vi "Test3.vi"() -> ()   [LabVIEW 2012]
uses:
  <vilib>/Rock Robotics/SystemInterfaces/DIO/FPGA_DIOChannel.ctl
  <vilib>/Rock Robotics/SystemInterfaces/DIO/FPGA_DIORelayChannel.ctl
  <vilib>/Rock Robotics/WPI/Solenoid/WPI_SolenoidChannel.ctl
  <vilib>/Rock Robotics/SystemInterfaces/Typedef/FPGA_TypedefSolenoidModule.ctl
  <vilib>/Rock Robotics/WPI/Solenoid/WPI_SolenoidValue.ctl
  <vilib>/Rock Robotics/WPI/Solenoid/WPI_SolenoidOpenDouble.vi
  <vilib>/Rock Robotics/WPI/Joystick/WPI_JoystickGetSetRefNum.vi
  <vilib>/Rock Robotics/WPI/Solenoid/WPI_SolenoidSetEnum.vi
panel:
  in  "TeleOp Elapsed Seconds":dbl
  in  "stop 2":bool
  in  "S On Time":dbl
  in  "S Off Time":dbl
  in  "stop":bool
  in  "Ready To Fire":bool
  out "Time Last Fired":dbl
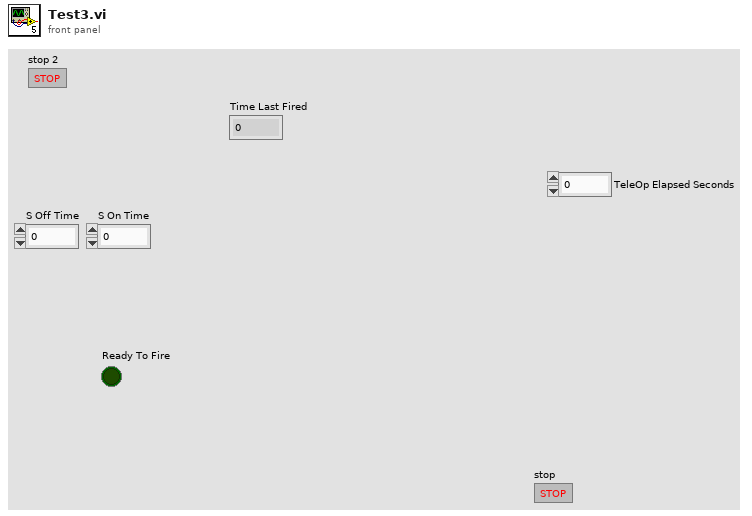
[diagram p1: front panel]
types:
  T1 = typedef "FPGA_DIORelayChannel.ctl" = enum8{"Relay 1", "Relay 2", "Relay 3", "Relay 4", "Relay 5", "Relay 6", "Relay 7", "Relay 8", "Invalid"}
  T2 = typedef "FPGA_DIOChannel.ctl" = enum8{"DIO 1", "DIO 2", "DIO 3", "DIO 4", "DIO 5", "DIO 6", "DIO 7", "DIO 8", "DIO 9", "DIO 10", "DIO 11", "DIO 12", "DIO 13", "DIO 14", "Invalid"}
  T3 = typedef "FPGA_TypedefSolenoidModule.ctl" = enum16{"Solenoid Module 1", "Solenoid Module 2"}
  T4 = typedef "WPI_SolenoidChannel.ctl" = enum8{"Solenoid 1", "Solenoid 2", "Solenoid 3", "Solenoid 4", "Solenoid 5", "Solenoid 6", "Solenoid 7", "Solenoid 8", "Invalid"}
  T5 = typedef "WPI_SolenoidValue.ctl" = enum16{"Off", "On", "Forward", "Reverse"}
  T6 = typedef "WPI_SolenoidDevRef.ctl" = cluster{"DevStatus":errorcluster, "Solenoid Module":T3, "Forward Solenoid Channel":T4, "Reverse Solenoid Channel":T4}
  T7 = typedef "WPI_JoystickDevRef.ctl" = cluster{"Device":T8}
  T8 = typedef "WPI_JoystickDeviceEnum.ctl" = enum16{"USB 1", "USB 2", "USB 3", "USB 4", "Kinect 1", "Kinect 2"}
  T9 = typedef "WPI_JoystickButtonState.ctl" = cluster{"Button 1":bool, "Button 2":bool, "Button 3":bool, "Button 4":bool, "Button 5":bool, "Button 6":bool, "Button 7":bool, "Button 8":bool, "Button 9":bool, "Button 10":bool, "Button 11":bool, "Button 12":bool}
  T10 = typedef "WPI_CompressorDevRef.ctl" = cluster{"DevStatus":errorcluster, "DigitalInputDevRef":T11, "RelayDevRef":T13}
  T11 = typedef "WPI_DigitalInputDevRef.ctl" = cluster{"DevStatus":errorcluster, "DIO Channel":T2, "Digital Module":T12}
  T12 = typedef "FPGA_TypedefDigitalModule.ctl" = enum16{"Digital Module 1", "Digital Module 2"}
  T13 = typedef "WPI_RelayDevRef.ctl" = cluster{"DevStatus":errorcluster, "Relay Channel":T1, "Digital Module":T12, "Relay Direction":T14}
  T14 = typedef "WPI_RelayDirection.ctl" = enum16{"Both directions", "Forward only", "Reverse only"}
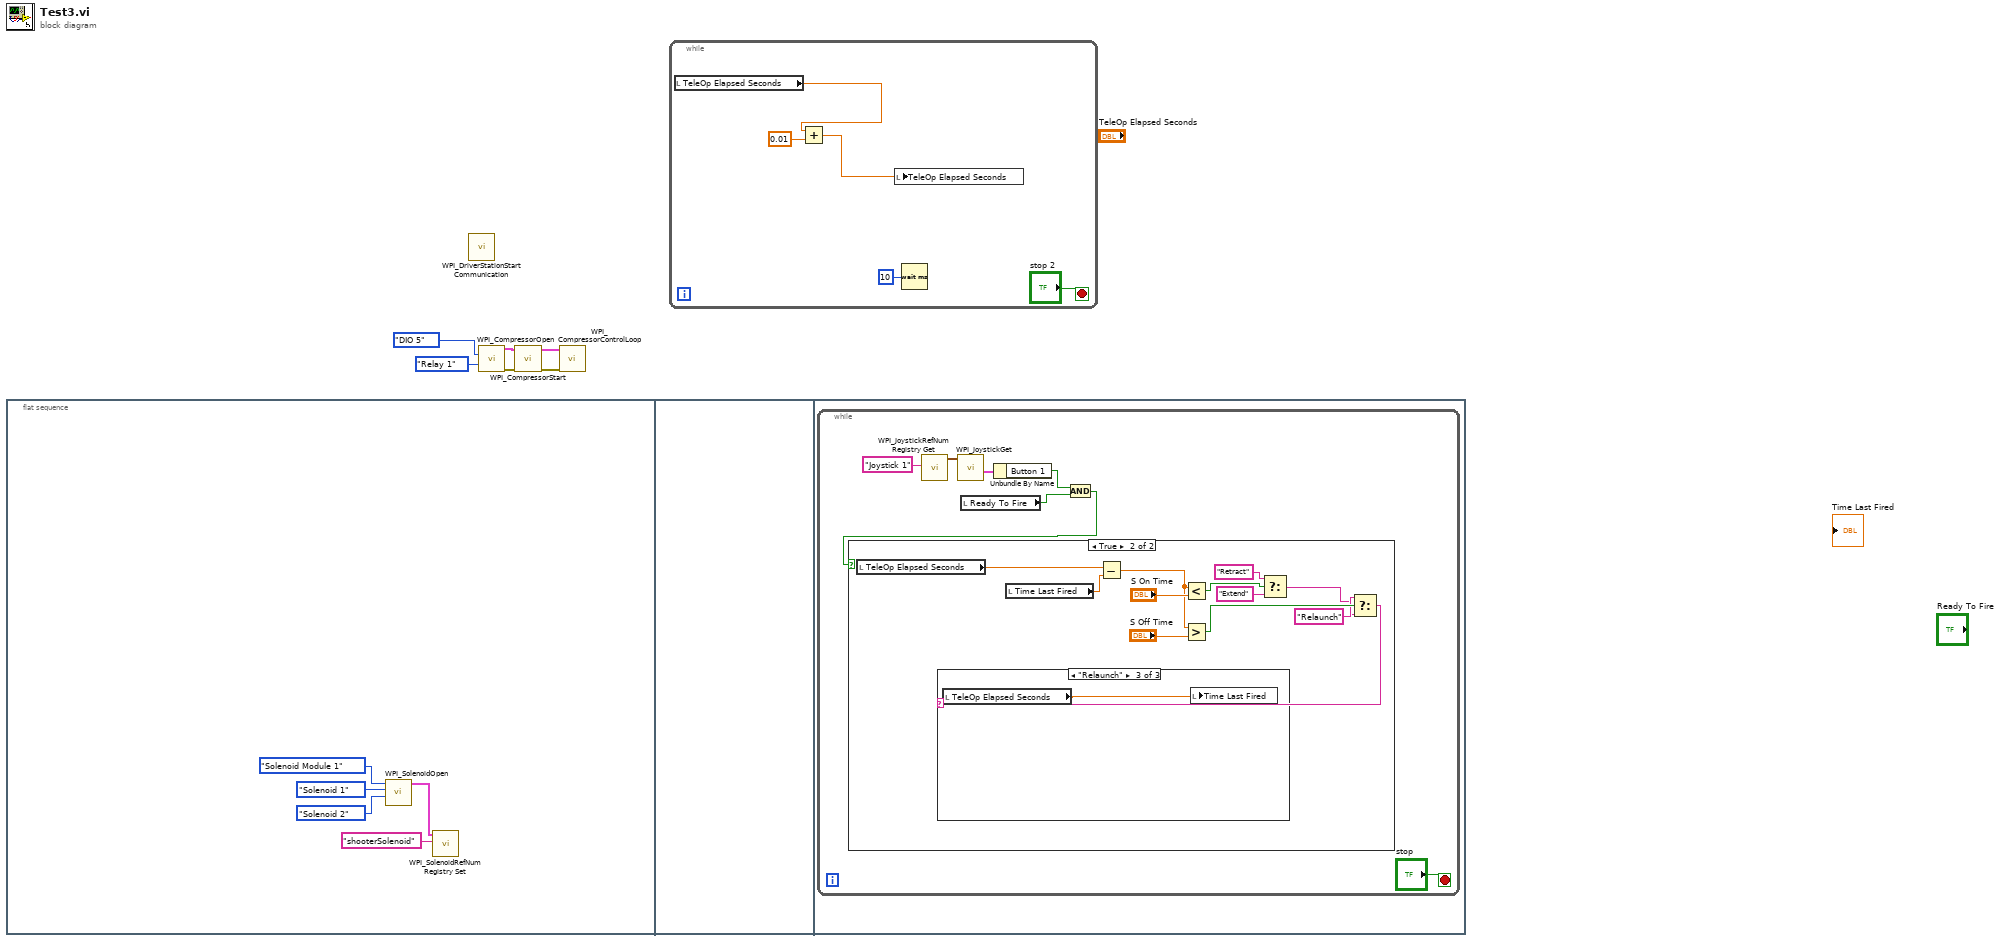
[diagram p0: block diagram]
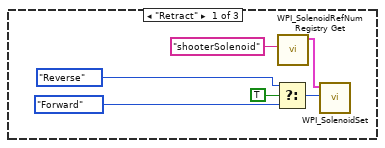
[diagram p3: hidden frame]
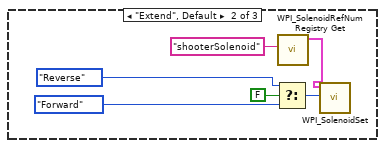
[diagram p4: hidden frame]
diagram:
  n1 = flat-sequence {
    frame #0 {
      n2 = call-poly <vilib>:"WPI_SolenoidOpen.vi"("Reverse Solenoid Channel"=WPI_SolenoidChannel."Solenoid 2", "Forward Solenoid Channel"=WPI_SolenoidChannel."Solenoid 1", "Solenoid Module (Module 1)"=FPGA_TypedefSolenoidModule."Solenoid Module 1") -> ("SolenoidDevRef"=w10:T6)  [unwired: 7 in, 1 out]
      n3 = call <vilib>:"WPI_SolenoidRefNum Registry Set.vi"("refnum name"="shooterSolenoid", "SolenoidDevRef"=w10) -> ()  [unwired: 8 in, 2 out]
    }
    frame #1 {
    }
    frame #2 {
      n4 = while {
        stop <- "stop" stop-if-true
        n5 = call <vilib>:"WPI_JoystickRefNum Registry Get.vi"("refnum name"="Joystick 1") -> ("JoystickDevRef"=w17:T7)  [unwired: 9 in, 1 out]
        n6 = call <vilib>:"WPI_JoystickGet.vi"("JoystickDevRef"=w17) -> ("Buttons"=w16:T9)  [unwired: 4 in, 2 out]
        n7 = local read "Ready To Fire"() -> (w14:bool)
        n8 = Unbundle By Name(w16) -> ("Button 1"=w12:bool)
        n9 = And(x=w12, y=w14) -> (x .and. y?=w15:bool)
        n10 = case shown="True" w15 {
          frame False {
          }
          frame True {
            n11 = local read "TeleOp Elapsed Seconds"() -> (w21:dbl)
            n12 = local read "Time Last Fired"() -> (w30:dbl)
            n13 = Subtract(x=w21, y=w30) -> (x-y=w24:dbl)
            n14 = Less?(x=w24, y="S On Time") -> (x < y?=w27:bool)
            n15 = Greater?(x=w24, y="S Off Time") -> (0:w22:bool)
            n16 = Select(t="Retract" ("f"), s=w27, f="Extend") -> (s? t:f=w19:string)
            n17 = Select(t="Relaunch" ("f"), s=w22, f=w19) -> (s? t:f=w28:string)
            n18 = case shown="\"Relaunch\"" w28 {
              frame "Retract" {
                n19 = Select(t=WPI_SolenoidValue."Reverse" ("Value"), s=TRUE, f=WPI_SolenoidValue."Forward" ("Value")) -> (s? t:f=w35:T5)
                n20 = call <vilib>:"WPI_SolenoidRefNum Registry Get.vi"("refnum name"="shooterSolenoid") -> ("SolenoidDevRef"=w31:T6)  [unwired: 9 in, 1 out]
                n21 = call-poly <vilib>:"WPI_SolenoidSet.vi"("Value"=w35, "SolenoidDevRef"=w31) -> ()  [unwired: 8 in, 2 out]
              }
              frame "Extend", Default {
                n22 = Select(t=WPI_SolenoidValue."Reverse" ("Value"), s=FALSE, f=WPI_SolenoidValue."Forward" ("Value")) -> (s? t:f=w41:T5)
                n23 = call <vilib>:"WPI_SolenoidRefNum Registry Get.vi"("refnum name"="shooterSolenoid") -> ("SolenoidDevRef"=w37:T6)  [unwired: 9 in, 1 out]
                n24 = call-poly <vilib>:"WPI_SolenoidSet.vi"("Value"=w41, "SolenoidDevRef"=w37) -> ()  [unwired: 8 in, 2 out]
              }
              frame "Relaunch" {
                n25 = local read "TeleOp Elapsed Seconds"() -> (w43:dbl)
                n26 = local write "Time Last Fired"(w43) -> ()
              }
            }
          }
        }
      }
    }
  }
  n27 = call <vilib>:"WPI_DriverStationStart Communication.vi"() -> ()  [unwired: 12 in]
  n28 = call <vilib>:"WPI_CompressorOpen.vi"("Pressure Switch DIO Channel"=FPGA_DIOChannel."DIO 5", "Relay Channel"=FPGA_DIORelayChannel."Relay 1") -> ("CompressorDevRef"=w3:T10, "error out"=w4:errorcluster)  [unwired: 12 in]
  n29 = call <vilib>:"WPI_CompressorStart.vi"("error in (no error)"=w4, "CompressorDevRef"=w3) -> ("error out"=w1:errorcluster, "CompressorDevRef"=w2:T10)  [unwired: 8 in]
  n30 = call <vilib>:"WPI_CompressorControlLoop.vi"("error in (no error)"=w1, "CompressorDevRef"=w2) -> ()  [unwired: 10 in]
  n31 = while {
    stop <- "stop 2" stop-if-true
    n32 = local read "TeleOp Elapsed Seconds"() -> (w45:dbl)
    n33 = Add(x=w45, y=0.01) -> (x+y=w46:dbl)
    n34 = local write "TeleOp Elapsed Seconds"(w46) -> ()
    n35 = Wait (ms)(milliseconds to wait=u32 10) -> ()  [unwired: 1 out]
  }
